vi "RESTful INI Regular Expression.vi"(8 "error in":errorcluster, 9 "offset (0)":i32, 11 "input string":string) -> (0 "error out":errorcluster, 1 "Offset of match":i32, 2 "whole match":string, 3 "dup input string":string, 4 "keyword":string, 5 "offset past match":i32)   [LabVIEW 2020]
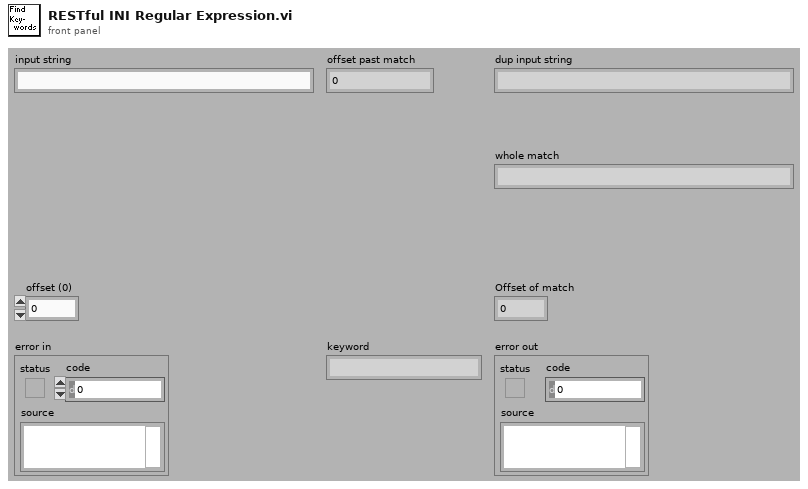
[diagram p1: front panel]
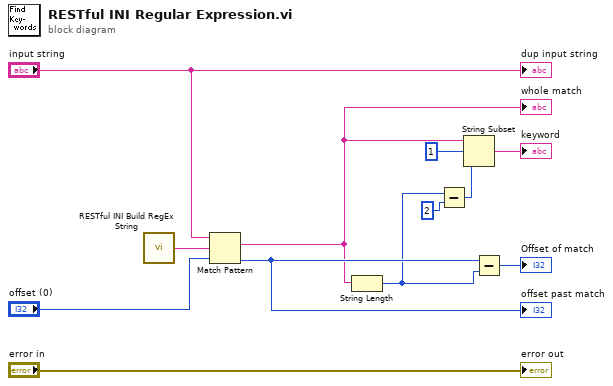
[diagram p0: block diagram]
diagram:
  n1 = call <vilib>:"RESTful INI Build RegEx String.vi"() -> ("keyword format (RegEx)"=w12:string)
  n2 = Match Pattern(string="input string", regular expression=w12, offset (0)="offset (0)") -> (match substring=w6:string, offset past match=w11:i32)  [unwired: 2 out]
  "offset past match" <- w11
  "whole match" <- w6
  n3 = String Length(string=w6) -> (length=w3:i32)
  n4 = Subtract(x=w3, y=2 ("offset (0)")) -> (x-y=w1:i32)
  n5 = String Subset(string=w6, offset (0)=1, length (rest)=w1) -> (substring=→"keyword":string)
  n6 = Subtract(x=w11, y=w3) -> (x-y=→"Offset of match":i32)
  "error out" <- "error in"
  "dup input string" <- "input string"
